vi "Generate Grid Plot.vi"(1 "Grid":set{cdb}(c389)) -> (0 "Grid Plot":cluster{cluster{i32, i32}[]}[](graph))   [LabVIEW 2020, in "AoC 2022.lvlib"]
uses:
  AoC 2022.lvlib
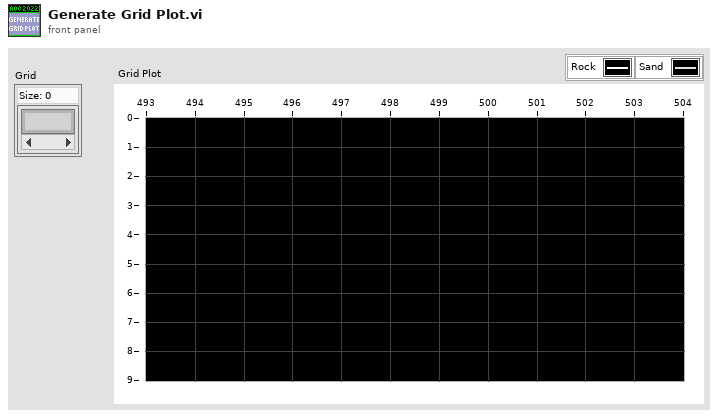
[diagram p1: front panel]
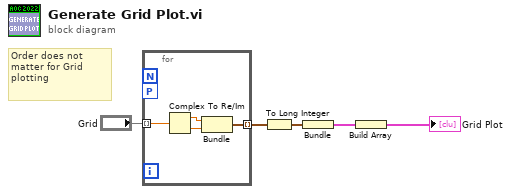
[diagram p0: block diagram]
diagram:
  # "Order does not matter for Grid plotting"
  n1 = for {
    tunnel: "Grid" -> [w9] mode=indexing
    tunnel: [w6] -> w4 mode=indexing
    workers-P: _ -> [_]
    n2 = Complex To Re/Im(x + iy=w9) -> (x=w8:dbl, y=w7:dbl)
    n3 = Bundle(w8, w7) -> (w6:cluster{dbl, dbl})  [unwired: 1 in]
  }
  n4 = To Long Integer(number=w4) -> (32bit integer=w3:cluster{i32, i32}[])
  n5 = Bundle(w3) -> (w2:cluster{cluster{i32, i32}[]})  [unwired: 1 in]
  n6 = Build Array(w2) -> (→"Grid Plot":cluster{cluster{i32, i32}[]}[])
